vi "Estimate New Pose.vi"(8 "Bot Angle (rad)":dbl, 9 "Linear Distance Travelled (mm)":dbl, 11 "Current Absolute Position":cluster{"X":dbl, "Y":dbl}) -> (3 "Updated Absolute Position":cluster{"X":dbl, "Y":dbl})   [LabVIEW 2017]
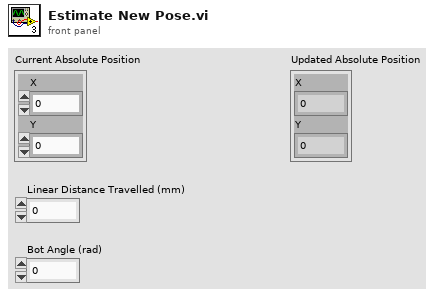
[diagram p1: front panel]
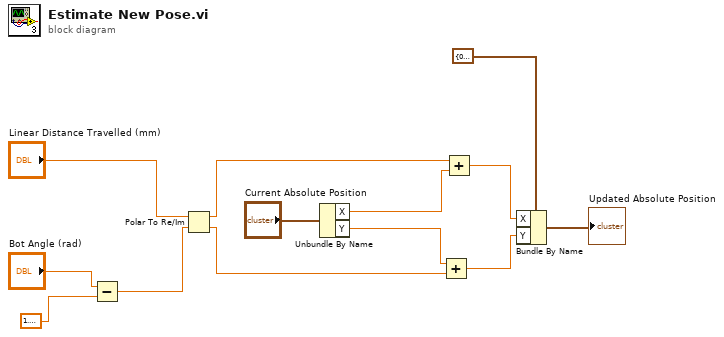
[diagram p0: block diagram]
diagram:
  n1 = Subtract(x="Bot Angle (rad)", y=1.5707963267948966) -> (x-y=w2:dbl)
  n2 = Polar To Re/Im(2:w2, 3:"Linear Distance Travelled (mm)") -> (0:w11:dbl, 1:w10:dbl)
  n3 = Unbundle By Name("Current Absolute Position") -> ("X"=w9:dbl, "Y"=w8:dbl)
  n4 = Add(x=w8, y=w11) -> (x+y=w6:dbl)
  n5 = Add(x=w10, y=w9) -> (x+y=w7:dbl)
  n6 = Bundle By Name(cluster=cluster{"X":dbl, "Y":dbl} {"X"=0.0, "Y"=0.0} ("Encoder-Estimated Absolute Position"), "X"=w7, "Y"=w6) -> (→"Updated Absolute Position":cluster{"X":dbl, "Y":dbl})
